vi "Invalid Response Parameters.vi"(7 "error source vi name":string, 8 "error in (no error)":errorcluster, 9 "actual parameters":T1, 10 "expected parameters":T1, 11 "Interface in":refnum<class "Interface.lvclass">) -> (0 "error out":errorcluster, 3 "Interface out":refnum<class "Interface.lvclass">)   [LabVIEW 2017, in "DSF Core.lvlib" / "Interface.lvclass"]
uses:
  Interface/Interface.lvclass
  Interface/RT FIFO Parameters.ctl
  Interface/Errors.ctl
  LabVIEW-Memory/Source/Static Errors.lvlib
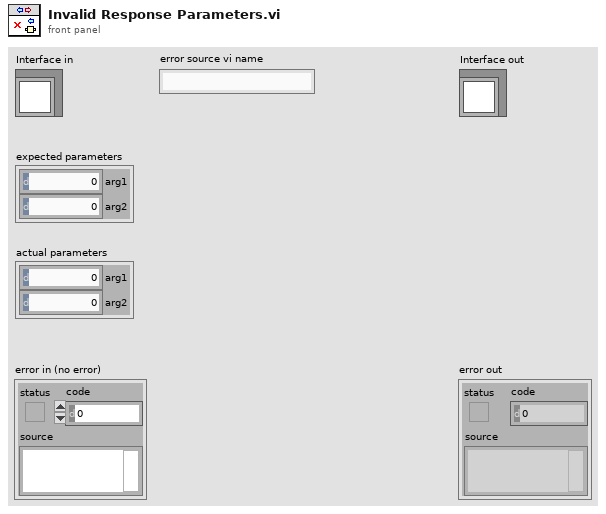
[diagram p1: front panel]
types:
  T1 = typedef "DSF Core.lvlib/Interface.lvclass/RT FIFO Parameters.ctl" = cluster{"arg1":u64, "arg2":u64}
  T2 = typedef "DSF Core.lvlib/Interface.lvclass/Errors.ctl" = enum16{"Command Timeout", "Response Timeout", "Error Timeout", "Invalid Response", "Invalid Response Parameters"}
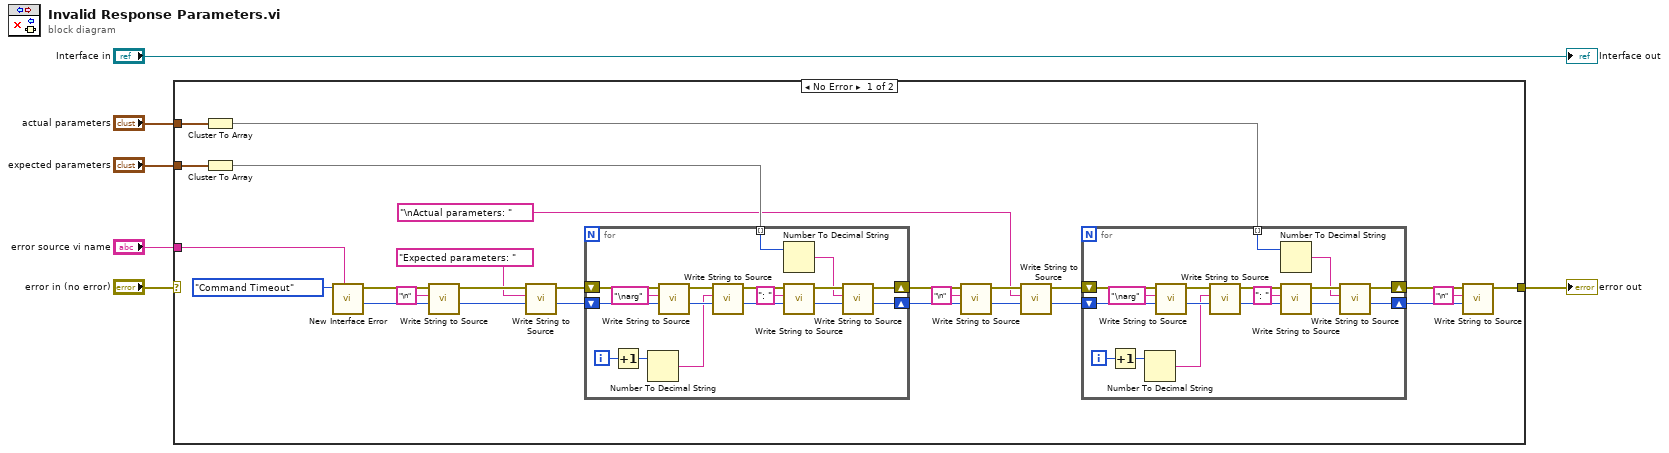
[diagram p0: block diagram]
diagram:
  n1 = case shown="No Error" "error in (no error)" {
    selector: "error in (no error)" -> [_ w67]
    tunnel: [w20 w67] -> w4
    tunnel: "error source vi name" -> [w32 _]
    tunnel: "actual parameters" -> [w18 _]
    tunnel: "expected parameters" -> [w19 _]
    frame No Error {
      n2 = Cluster To Array(cluster=w18) -> (array=w8:u64[])
      n3 = Cluster To Array(cluster=w19) -> (array=w17:u64[])
      n4 = call "New Interface Error.vi"("error source vi name"=w32, "error"=Errors."Command Timeout") -> ("new offset"=w30:i32, "error out"=w31:errorcluster)  [unwired: 8 in]
      n5 = call "Write String to Source.vi"("offset"=w30, "string"="\n", "error in"=w31) -> ("new offset"=w27:i32, "error out"=w28:errorcluster)  [unwired: 7 in]
      n6 = call "Write String to Source.vi"("offset"=w27, "string"="Expected parameters: ", "error in"=w28) -> ("new offset"=w26:i32, "error out"=w25:errorcluster)  [unwired: 7 in]
      n7 = for {
        shift-right: [w33] -> w14
        shift-left: w26 -> [w49]
        shift-right: [w34] -> w15
        shift-left: w25 -> [w48]
        tunnel: w17 -> [w38] mode=indexing
        i -> [w44]
        n8 = Increment(x=w44) -> (x+1=w45:i32)
        n9 = Number To Decimal String(number=w45) -> (decimal integer string=w42:string)  [unwired: 1 in]
        n10 = call "Write String to Source.vi"("offset"=w49, "string"="\narg", "error in"=w48) -> ("new offset"=w43:i32, "error out"=w47:errorcluster)  [unwired: 7 in]
        n11 = call "Write String to Source.vi"("offset"=w43, "string"=w42, "error in"=w47) -> ("new offset"=w40:i32, "error out"=w41:errorcluster)  [unwired: 7 in]
        n12 = Number To Decimal String(number=w38) -> (decimal integer string=w35:string)  [unwired: 1 in]
        n13 = call "Write String to Source.vi"("offset"=w40, "string"=": ", "error in"=w41) -> ("new offset"=w36:i32, "error out"=w37:errorcluster)  [unwired: 7 in]
        n14 = call "Write String to Source.vi"("offset"=w36, "string"=w35, "error in"=w37) -> ("new offset"=w33:i32, "error out"=w34:errorcluster)  [unwired: 7 in]
      }
      n15 = call "Write String to Source.vi"("offset"=w14, "string"="\n", "error in"=w15) -> ("new offset"=w12:i32, "error out"=w13:errorcluster)  [unwired: 7 in]
      n16 = call "Write String to Source.vi"("offset"=w12, "string"="\nActual parameters: ", "error in"=w13) -> ("new offset"=w22:i32, "error out"=w23:errorcluster)  [unwired: 7 in]
      n17 = for {
        shift-right: [w50] -> w9
        shift-left: w22 -> [w66]
        shift-right: [w51] -> w10
        shift-left: w23 -> [w65]
        tunnel: w8 -> [w55] mode=indexing
        i -> [w61]
        n18 = Increment(x=w61) -> (x+1=w62:i32)
        n19 = Number To Decimal String(number=w62) -> (decimal integer string=w59:string)  [unwired: 1 in]
        n20 = call "Write String to Source.vi"("offset"=w66, "string"="\narg", "error in"=w65) -> ("new offset"=w60:i32, "error out"=w64:errorcluster)  [unwired: 7 in]
        n21 = call "Write String to Source.vi"("offset"=w60, "string"=w59, "error in"=w64) -> ("new offset"=w57:i32, "error out"=w58:errorcluster)  [unwired: 7 in]
        n22 = Number To Decimal String(number=w55) -> (decimal integer string=w52:string)  [unwired: 1 in]
        n23 = call "Write String to Source.vi"("offset"=w57, "string"=": ", "error in"=w58) -> ("new offset"=w53:i32, "error out"=w54:errorcluster)  [unwired: 7 in]
        n24 = call "Write String to Source.vi"("offset"=w53, "string"=w52, "error in"=w54) -> ("new offset"=w50:i32, "error out"=w51:errorcluster)  [unwired: 7 in]
      }
      n25 = call "Write String to Source.vi"("offset"=w9, "string"="\n", "error in"=w10) -> ("error out"=w20:errorcluster)  [unwired: 7 in, 1 out]
    }
    frame Error {
    }
  }
  "error out" <- w4
  "Interface out" <- "Interface in"
